vi "Append Test Suites Result.vi"(8 "error in (no error)":errorcluster, 11 "Plain Text Report In":refnum<class "Plain Text Report.lvclass">) -> (0 "error out":errorcluster, 3 "Plain Text Report Out":refnum<class "Plain Text Report.lvclass">)   [LabVIEW 2020, in "Plain Text Report.lvclass"]
uses:
  Plain Text Report.lvclass
  Test Report/Test Report.lvclass
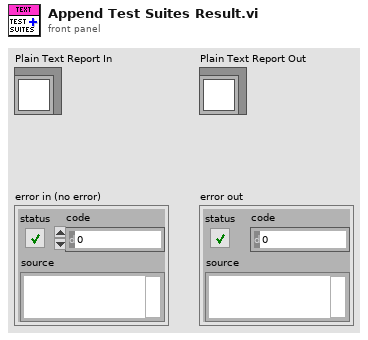
[diagram p1: front panel]
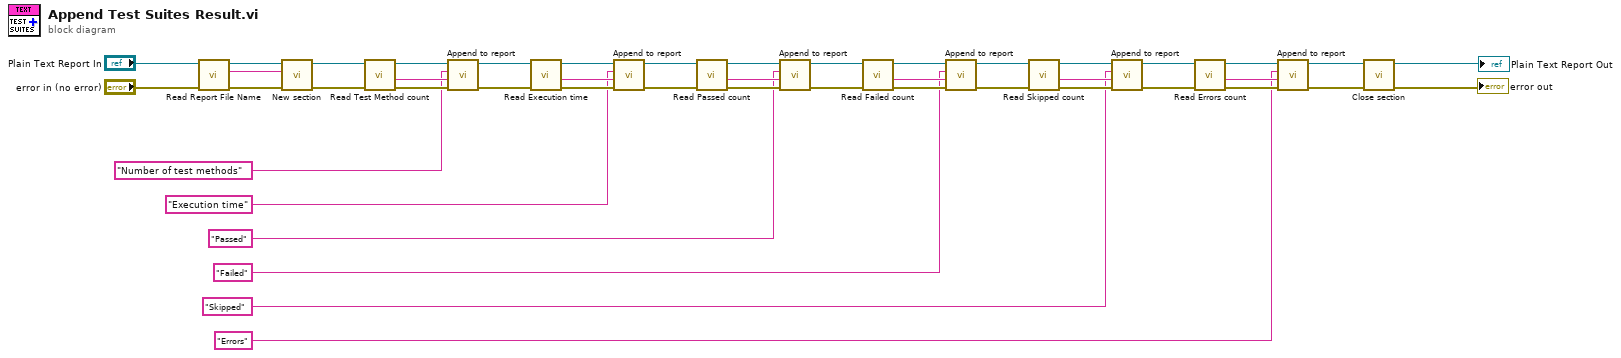
[diagram p0: block diagram]
diagram:
  n1 = call-dynamic "Read Report File Name.vi"("error in (no error)"="error in (no error)", "Plain Text Report In"="Plain Text Report In") -> ("error out"=w6:errorcluster, "Report Name"=w5:string, "Plain Text Report Out"=w9:refnum<class "Plain Text Report.lvclass">)  [unwired: 6 in, 1 out]
  n2 = call "New section.vi"("error in (no error)"=w6, "Section name"=w5, "Plain Text Report In"=w9) -> ("error out"=w7:errorcluster, "Plain Text Report Out"=w8:refnum<class "Plain Text Report.lvclass">)  [unwired: 7 in]
  n3 = call "Read Test Method count.vi"("error in (no error)"=w7, "Report In"=w8) -> ("error out"=w40:errorcluster, "Test Method count string"=w37:string, "Report Out"=w41:refnum<class "Plain Text Report.lvclass">)  [unwired: 6 in, 1 out]
  n4 = call "Append to report.vi"("error in (no error)"=w40, "Value"=w37, "Key"="Number of test methods" ("Name"), "Plain Text Report In"=w41) -> ("error out"=w26:errorcluster, "Plain Text Report Out"=w27:refnum<class "Plain Text Report.lvclass">)  [unwired: 6 in]
  n5 = call "Read Execution time.vi"("error in (no error)"=w26, "Report In"=w27) -> ("error out"=w35:errorcluster, "Execution time string"=w34:string, "Report Out"=w36:refnum<class "Plain Text Report.lvclass">)  [unwired: 6 in, 1 out]
  n6 = call "Append to report.vi"("error in (no error)"=w35, "Value"=w34, "Key"="Execution time" ("Name"), "Plain Text Report In"=w36) -> ("error out"=w24:errorcluster, "Plain Text Report Out"=w25:refnum<class "Plain Text Report.lvclass">)  [unwired: 6 in]
  n7 = call "Read Passed count.vi"("error in (no error)"=w24, "Report In"=w25) -> ("error out"=w33:errorcluster, "Passed count string"=w31:string, "Report Out"=w32:refnum<class "Plain Text Report.lvclass">)  [unwired: 6 in, 1 out]
  n8 = call "Append to report.vi"("error in (no error)"=w33, "Value"=w31, "Key"="Passed" ("Name"), "Plain Text Report In"=w32) -> ("error out"=w22:errorcluster, "Plain Text Report Out"=w23:refnum<class "Plain Text Report.lvclass">)  [unwired: 6 in]
  n9 = call "Read Failed count.vi"("error in (no error)"=w22, "Report In"=w23) -> ("error out"=w42:errorcluster, "Failed count string"=w38:string, "Report Out"=w43:refnum<class "Plain Text Report.lvclass">)  [unwired: 6 in, 1 out]
  n10 = call "Append to report.vi"("error in (no error)"=w42, "Value"=w38, "Key"="Failed" ("Name"), "Plain Text Report In"=w43) -> ("error out"=w20:errorcluster, "Plain Text Report Out"=w21:refnum<class "Plain Text Report.lvclass">)  [unwired: 6 in]
  n11 = call "Read Skipped count.vi"("error in (no error)"=w20, "Report In"=w21) -> ("error out"=w30:errorcluster, "Skipped count string"=w28:string, "Report Out"=w29:refnum<class "Plain Text Report.lvclass">)  [unwired: 6 in, 1 out]
  n12 = call "Append to report.vi"("error in (no error)"=w30, "Value"=w28, "Key"="Skipped" ("Name"), "Plain Text Report In"=w29) -> ("error out"=w18:errorcluster, "Plain Text Report Out"=w19:refnum<class "Plain Text Report.lvclass">)  [unwired: 6 in]
  n13 = call "Read Errors count.vi"("error in (no error)"=w18, "Report In"=w19) -> ("error out"=w44:errorcluster, "Errors count string"=w39:string, "Report Out"=w45:refnum<class "Plain Text Report.lvclass">)  [unwired: 6 in, 1 out]
  n14 = call "Append to report.vi"("error in (no error)"=w44, "Value"=w39, "Key"="Errors" ("Name"), "Plain Text Report In"=w45) -> ("error out"=w2:errorcluster, "Plain Text Report Out"=w4:refnum<class "Plain Text Report.lvclass">)  [unwired: 6 in]
  n15 = call "Close section.vi"("error in (no error)"=w2, "Plain Text Report In"=w4) -> ("error out"=→"error out":errorcluster, "Plain Text Report Out"=→"Plain Text Report Out":refnum<class "Plain Text Report.lvclass">)  [unwired: 8 in]
